vi "Verify is full array.vi"(8 "error in (no error)":errorcluster, 10 "Value":string[][](array[string]), 11 "Array in":string[](array[string])) -> (0 "error out":errorcluster, 3 "Data Salida":string[][](array[string]))   [LabVIEW 2018]
uses:
  Controles/Lista Modulos.ctl
  Comunicacion/Mensajes.lvlib
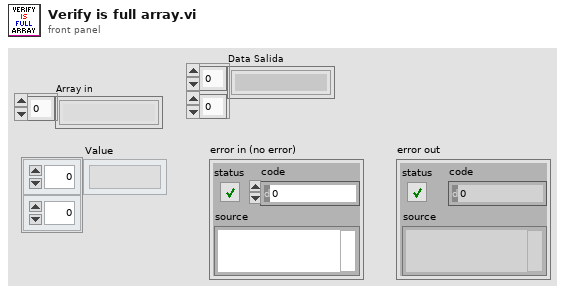
[diagram p1: front panel]
types:
  T1 = typedef "Lista Modulos.ctl" = enum16{"Math", "Error", "Front", "Database", "Nuevos items"}
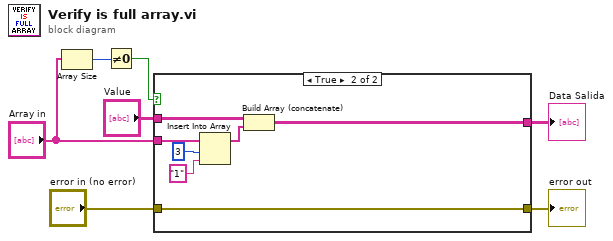
[diagram p0: block diagram]
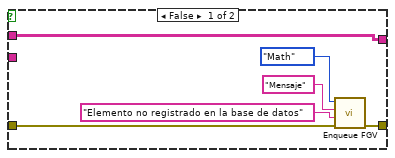
[diagram p2: hidden frame]
diagram:
  n1 = Array Size(array="Array in") -> (size(s)=w6:i32)
  n2 = Not Equal To 0?(x=w6) -> (x != 0?=w5:bool)
  n3 = case shown="True" w5 {
    tunnel: [w8 w14] -> w1
    tunnel: "Array in" -> [_ w18]
    tunnel: "error in (no error)" -> [w10 w17]
    tunnel: [w9 w17] -> w3
    tunnel: "Value" -> [w8 w16]
    frame False {
      n4 = call "Enqueue FGV.vi"("error in (no error)"=w10, "Dato"="Elemento no registrado en la base de datos" ("Mensaje"), "Mensaje"="Mensaje", "Modulo a obtener"=Lista_Modulos."Math") -> ("error out"=w9:errorcluster)  [unwired: 7 in]
    }
    frame True {
      n5 = Insert Into Array(array=w18, index=3, new element="1" ("new element/subarray")) -> (w15:string[])
      n6 = Build Array (concatenate)(w16, w15) -> (w14:string[][])
    }
  }
  "error out" <- w3
  "Data Salida" <- w1
